vi "Storage.vi"(11 "Overlay Filter in":refnum<class "Overlay Filter.lvclass">) -> (2 "Storage":refnum<class "Config Storage.lvclass">)   [LabVIEW 2020, in "CDM-Config.lvlib" / "Overlay Filter.lvclass"]
uses:
  Overlay Filter.lvclass
  Config Storage/Config Storage.lvclass
  Overlay Filter.lvclass/Overlay Filter.ctl
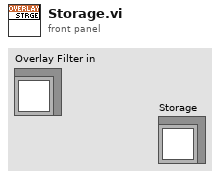
[diagram p1: front panel]
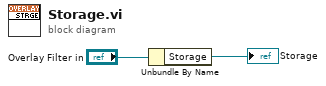
[diagram p0: block diagram]
diagram:
  n1 = Unbundle By Name("Overlay Filter in") -> ("Storage"=→"Storage":refnum<class "Config Storage.lvclass">)
